vi "Area of triangle.vi"() -> ()   [LabVIEW 2022 SP3]
panel:
  out "Numeric":dbl
  out "Valid Triangle":bool
  in  "Side B (cm)":dbl
  in  "Side C (cm)":dbl
  in  "Side A (cm)":dbl
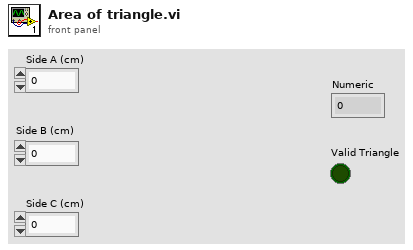
[diagram p1: front panel]
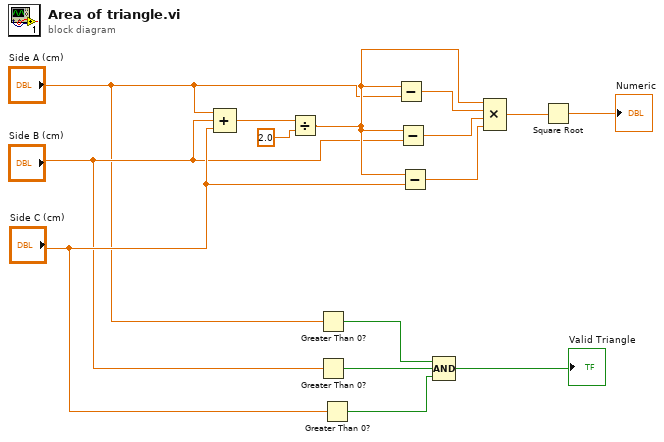
[diagram p0: block diagram]
diagram:
  n1 = Compound Arithmetic op=ADD("Side A (cm)", "Side B (cm)", "Side C (cm)") -> (w11:dbl)
  n2 = Divide(x=w11, y=2.0) -> (x/y=w10:dbl)
  n3 = Greater Than 0?(x="Side A (cm)") -> (x > 0?=w15:bool)
  n4 = Greater Than 0?(x="Side B (cm)") -> (x > 0?=w14:bool)
  n5 = Greater Than 0?(x="Side C (cm)") -> (x > 0?=w5:bool)
  n6 = Subtract(x=w10, y="Side A (cm)") -> (x-y=w9:dbl)
  n7 = Subtract(x=w10, y="Side B (cm)") -> (x-y=w7:dbl)
  n8 = Subtract(x=w10, y="Side C (cm)") -> (x-y=w8:dbl)
  n9 = Compound Arithmetic op=AND(w15, w14, w5) -> (→"Valid Triangle":bool)
  n10 = Compound Arithmetic op=MULTIPLY(w10, w9, w7, w8) -> (w6:dbl)
  n11 = Square Root(x=w6) -> (sqrt(x)=→"Numeric":dbl)
